vi "Delete from Array (Value[]).vi"(8 "error in (no error)":errorcluster, 9 "index":i32, 10 "length":i32, 11 "JSON Array In":refnum<class "JSON Value.lvclass">) -> (0 "error out":errorcluster, 1 "deleted portion":refnum<class "JSON Value.lvclass">[](array[class]), 3 "JSON Array w/ subset deleted":refnum<class "JSON Value.lvclass">)   [LabVIEW 2016, in "JSON Value.lvclass"]
doc: "Deletes an element or subarray from a JSON array of length elements starting at index. Returns the edited array in array w/ subset deleted and the deleted element or subarray in deleted portion."
uses:
  JSON Value.lvclass
  JSON Value.lvclass/JSON Value.ctl
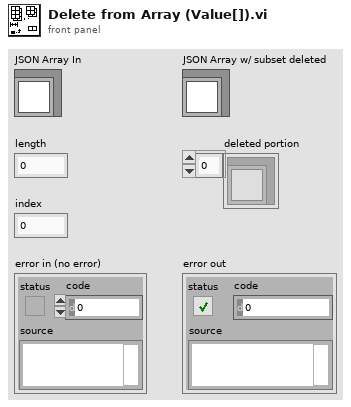
[diagram p1: front panel]
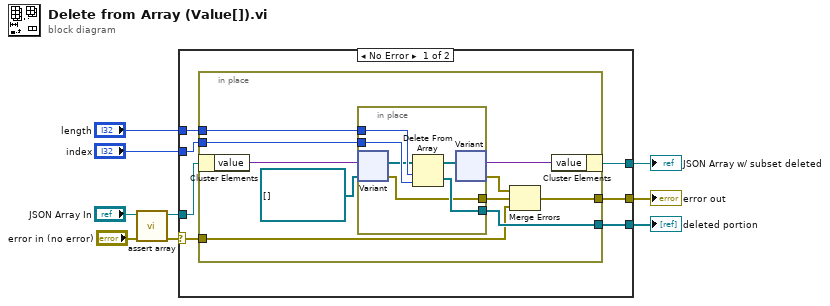
[diagram p0: block diagram]
diagram:
  n1 = call "assert array.vi"("error in (no error)"="error in (no error)", "JSON Value in"="JSON Array In") -> ("error out"=w3:errorcluster, "JSON Value out"=w4:refnum<class "JSON Value.lvclass">)  [unwired: 8 in]
  n2 = case shown="No Error" w3 {
    selector: w3 -> [w11 w33]
    tunnel: "index" -> [w16 _]
    tunnel: [w15 w34] -> w7
    tunnel: "length" -> [w14 _]
    tunnel: [w13 _] -> w5
    tunnel: w4 -> [w12 w34]
    tunnel: [w10 w33] -> w2
    frame No Error {
      n3 = in-place {
        in-place-border: w16 -> [w26]
        in-place-border: [w25] -> w13
        in-place-border: w14 -> [w24]
        in-place-border: w11 -> [w18]
        in-place-border: [w17] -> w10
        n4 = in-place-cluster #1(w12) -> ("value"=w22:variant)
        n5 = in-place {
          in-place-border: w26 -> [w32]
          in-place-border: [w31] -> w25
          in-place-border: w24 -> [w30]
          in-place-border: [w27] -> w19
          n6 = in-place-variant #2(w22, refnum<class "JSON Value.lvclass">[] [] ("JSON Array In")) -> (w29:refnum<class "JSON Value.lvclass">[], w27:errorcluster)
          n7 = Delete From Array(array=w29, length=w30, index=w32) -> (deleted portion=w31:refnum<class "JSON Value.lvclass">[], array with subset deleted=w28:refnum<class "JSON Value.lvclass">[])
          n8 = in-place-variant #2(w28) -> (w21:variant, w20:errorcluster)
        }
        n9 = Merge Errors(w20, w19, w18) -> (w17:errorcluster)
        n10 = in-place-cluster #1("value"=w21) -> (w15:refnum<class "JSON Value.lvclass">)
      }
    }
    frame Error {
    }
  }
  "JSON Array w/ subset deleted" <- w7
  "deleted portion" <- w5
  "error out" <- w2
